vi "校准参数写入.vi"(8 "error in":errorcluster caption="错误输入", 9 "截距":i32 format="%.0x", 10 "斜率":i32 format="%.0x", 11 "Channel":u16=81 format="%.0x") -> (0 "error out":errorcluster caption="错误输出", 3 "Channel out":u16)   [LabVIEW 2020]
uses:
  D/Program Files (x86)/National Instruments/LabVIEW 2020/user.lib/PCANBasic/PCANBasic.lvlib
panel:
  out "function return 2":u32 format="%.0x"
  out "function return":u32 format="%.0x"
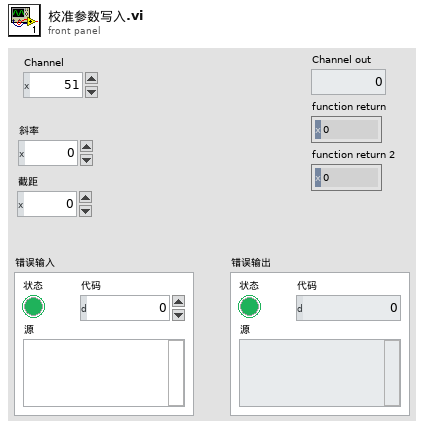
[diagram p1: front panel]
types:
  T1 = cluster{"ID":u32, "MSGTYPE":u8, "DLC":u8, "DATA[0]":u8, "DATA[1]":u8, "DATA[2]":u8, "DATA[3]":u8, "DATA[4]":u8, "DATA[5]":u8, "DATA[6]":u8, "DATA[7]":u8, "DATA[8]":u8, "DATA[9]":u8, "DATA[10]":u8, "DATA[11]":u8, "DATA[12]":u8, "DATA[13]":u8, "DATA[14]":u8, "DATA[15]":u8, "DATA[16]":u8, "DATA[17]":u8, "DATA[18]":u8, "DATA[19]":u8, "DATA[20]":u8, "DATA[21]":u8, "DATA[22]":u8, "DATA[23]":u8, "DATA[24]":u8, "DATA[25]":u8, "DATA[26]":u8, "DATA[27]":u8, "DATA[28]":u8, "DATA[29]":u8, "DATA[30]":u8, "DATA[31]":u8, "DATA[32]":u8, "DATA[33]":u8, "DATA[34]":u8, "DATA[35]":u8, "DATA[36]":u8, "DATA[37]":u8, "DATA[38]":u8, "DATA[39]":u8, "DATA[40]":u8, "DATA[41]":u8, "DATA[42]":u8, "DATA[43]":u8, "DATA[44]":u8, "DATA[45]":u8, "DATA[46]":u8, "DATA[47]":u8, "DATA[48]":u8, "DATA[49]":u8, "DATA[50]":u8, "DATA[51]":u8, "DATA[52]":u8, "DATA[53]":u8, "DATA[54]":u8, "DATA[55]":u8, "DATA[56]":u8, "DATA[57]":u8, "DATA[58]":u8, "DATA[59]":u8, "DATA[60]":u8, "DATA[61]":u8, "DATA[62]":u8, "DATA[63]":u8}
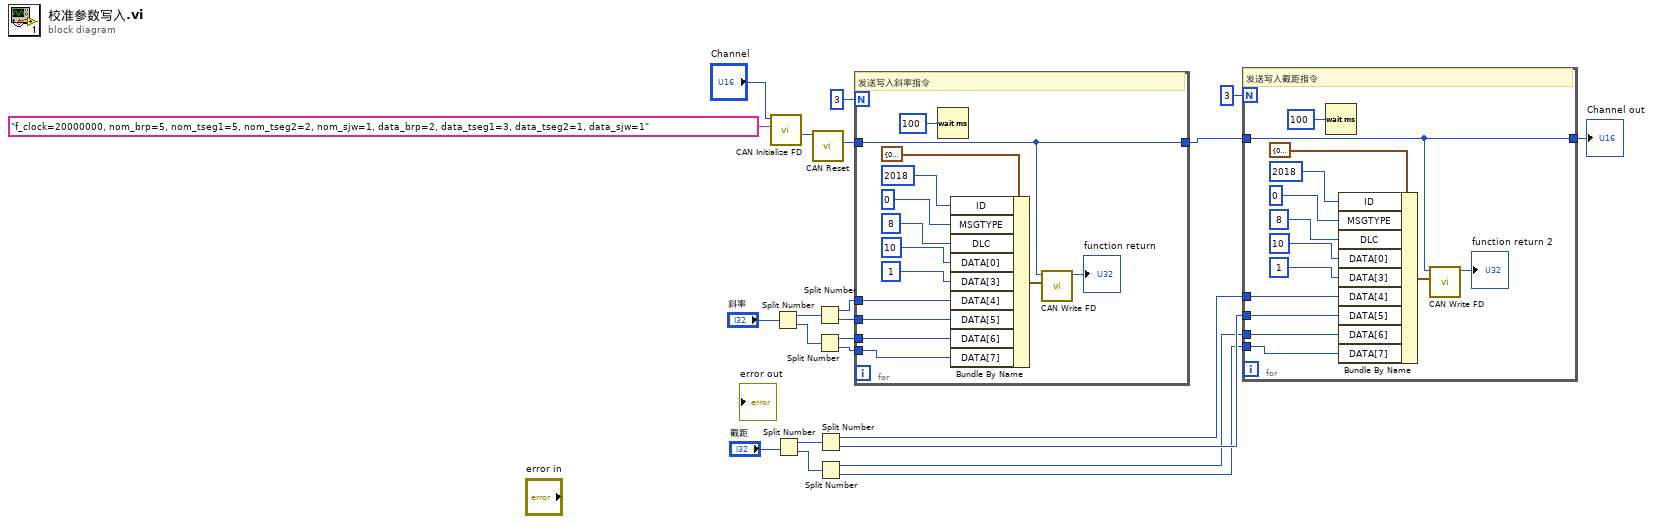
[diagram p0: block diagram]
diagram:
  n1 = call "CAN Initialize FD.vi"("BitrateFD"="f_clock=20000000, nom_brp=5, nom_tseg1=5, nom_tseg2=2, nom_sjw=1, data_brp=2, data_tseg1=3, data_tseg2=1, data_sjw=1", "Channel"="Channel") -> ("Channel out"=w19:u16)  [unwired: 7 in, 2 out]
  n2 = Split Number(x="斜率") -> (hi(x)=w16:u16, lo(x)=w15:u16)
  n3 = Split Number(x="截距") -> (hi(x)=w9:u16, lo(x)=w10:u16)
  n4 = call "CAN Reset.vi"("Channel in"=w19) -> ("Channel out"=w18:u16)  [unwired: 9 in, 1 out]
  n5 = Split Number(x=w16) -> (hi(x)=w14:u8, lo(x)=w13:u8)
  n6 = Split Number(x=w15) -> (hi(x)=w12:u8, lo(x)=w11:u8)
  n7 = Split Number(x=w9) -> (hi(x)=w7:u8, lo(x)=w6:u8)
  n8 = Split Number(x=w10) -> (hi(x)=w5:u8, lo(x)=w4:u8)
  n9 = for {
    N: 3 -> [_]
    tunnel: w18 -> [w33]
    tunnel: [w33] -> w3
    tunnel: w14 -> [w26]
    tunnel: w13 -> [w25]
    tunnel: w12 -> [w24]
    tunnel: w11 -> [w23]
    # "发送写入斜率指令"
    n10 = Wait (ms)(milliseconds to wait=u32 100 ("等待时间（毫秒）")) -> ()  [unwired: 1 out]
    n11 = Bundle By Name(cluster=T1 {"ID"=0, "MSGTYPE"=0, "DLC"=0, "DATA[0]"=0, "DATA[1]"=0, "DATA[2]"=0, "DATA[3]"=0, "DATA[4]"=0, "DATA[5]"=0, "DATA[6]"=0, "DATA[7]"=0, "DATA[8]"=0, "DATA[9]"=0, "DATA[10]"=0, "DATA[11]"=0, "DATA[12]"=0, "DATA[13]"=0, "DATA[14]"=0, "DATA[15]"=0, "DATA[16]"=0, "DATA[17]"=0, "DATA[18]"=0, "DATA[19]"=0, "DATA[20]"=0, "DATA[21]"=0, "DATA[22]"=0, "DATA[23]"=0, "DATA[24]"=0, "DATA[25]"=0, "DATA[26]"=0, "DATA[27]"=0, "DATA[28]"=0, "DATA[29]"=0, "DATA[30]"=0, "DATA[31]"=0, "DATA[32]"=0, "DATA[33]"=0, "DATA[34]"=0, "DATA[35]"=0, "DATA[36]"=0, "DATA[37]"=0, "DATA[38]"=0, "DATA[39]"=0, "DATA[40]"=0, "DATA[41]"=0, "DATA[42]"=0, "DATA[43]"=0, "DATA[44]"=0, "DATA[45]"=0, "DATA[46]"=0, "DATA[47]"=0, "DATA[48]"=0, "DATA[49]"=0, "DATA[50]"=0, "DATA[51]"=0, "DATA[52]"=0, "DATA[53]"=0, "DATA[54]"=0, "DATA[55]"=0, "DATA[56]"=0, "DATA[57]"=0, "DATA[58]"=0, "DATA[59]"=0, "DATA[60]"=0, "DATA[61]"=0, "DATA[62]"=0, "DATA[63]"=0} ("MessageBuffer"), "ID"=u32 2018, "MSGTYPE"=u8 0, "DLC"=u8 8 ("ID"), "DATA[0]"=u8 10 ("ID"), "DATA[3]"=u8 1, "DATA[4]"=w26, "DATA[5]"=w25, "DATA[6]"=w24, "DATA[7]"=w23) -> (w27:T1)
    n12 = call "CAN Write FD.vi"("MessageBuffer"=w27, "Channel"=w33) -> ("function return"=→"function return":u32)  [unwired: 7 in, 2 out]
  }
  n13 = for {
    N: 3 -> [_]
    tunnel: w3 -> [w47]
    tunnel: [w47] -> w1
    tunnel: w7 -> [w40]
    tunnel: w6 -> [w39]
    tunnel: w5 -> [w38]
    tunnel: w4 -> [w37]
    # "发送写入截距指令"
    n14 = Wait (ms)(milliseconds to wait=u32 100 ("等待时间（毫秒）")) -> ()  [unwired: 1 out]
    n15 = Bundle By Name(cluster=T1 {"ID"=0, "MSGTYPE"=0, "DLC"=0, "DATA[0]"=0, "DATA[1]"=0, "DATA[2]"=0, "DATA[3]"=0, "DATA[4]"=0, "DATA[5]"=0, "DATA[6]"=0, "DATA[7]"=0, "DATA[8]"=0, "DATA[9]"=0, "DATA[10]"=0, "DATA[11]"=0, "DATA[12]"=0, "DATA[13]"=0, "DATA[14]"=0, "DATA[15]"=0, "DATA[16]"=0, "DATA[17]"=0, "DATA[18]"=0, "DATA[19]"=0, "DATA[20]"=0, "DATA[21]"=0, "DATA[22]"=0, "DATA[23]"=0, "DATA[24]"=0, "DATA[25]"=0, "DATA[26]"=0, "DATA[27]"=0, "DATA[28]"=0, "DATA[29]"=0, "DATA[30]"=0, "DATA[31]"=0, "DATA[32]"=0, "DATA[33]"=0, "DATA[34]"=0, "DATA[35]"=0, "DATA[36]"=0, "DATA[37]"=0, "DATA[38]"=0, "DATA[39]"=0, "DATA[40]"=0, "DATA[41]"=0, "DATA[42]"=0, "DATA[43]"=0, "DATA[44]"=0, "DATA[45]"=0, "DATA[46]"=0, "DATA[47]"=0, "DATA[48]"=0, "DATA[49]"=0, "DATA[50]"=0, "DATA[51]"=0, "DATA[52]"=0, "DATA[53]"=0, "DATA[54]"=0, "DATA[55]"=0, "DATA[56]"=0, "DATA[57]"=0, "DATA[58]"=0, "DATA[59]"=0, "DATA[60]"=0, "DATA[61]"=0, "DATA[62]"=0, "DATA[63]"=0} ("MessageBuffer"), "ID"=u32 2018, "MSGTYPE"=u8 0, "DLC"=u8 8 ("ID"), "DATA[0]"=u8 10 ("ID"), "DATA[3]"=u8 1, "DATA[4]"=w40, "DATA[5]"=w39, "DATA[6]"=w38, "DATA[7]"=w37) -> (w41:T1)
    n16 = call "CAN Write FD.vi"("MessageBuffer"=w41, "Channel"=w47) -> ("function return"=→"function return 2":u32)  [unwired: 7 in, 2 out]
  }
  "Channel out" <- w1
